vi "CAL-Interp (Fs, Npts).vi"(0 "Frequency (Hz)":dbl[](array[numeric]), 5 "Magnitude (dB)":dbl[](array[numeric]), 7 "Phase (degrees)":dbl[](array[numeric]), 9 "Fs (Hz)":dbl, 11 "Npts":i32) -> (4 "Interp Freq (Hz)":dbl[](array[numeric]), 6 "Interp Magnitude (dB)":dbl[](array[numeric]), 8 "Interp Phase (degrees)":dbl[](array[numeric]), 15 "Interp z":cdb[](array[numeric]))   [LabVIEW 2020]
uses:
  epl-vi-lib/Utility VIs/Math VIs/LinSpace (x0-dx-npts).vi
  918d1905-b6a0-4792-ae90-c7ddb557a04e.vi
  134e58aa-5bf1-43ce-a1c6-9a5bd50e3390.vi
  e1cc8427-bc3c-4687-9115-91c34d18d393.vi
  <vilib>/gmath/NI_Gmath.lvlib
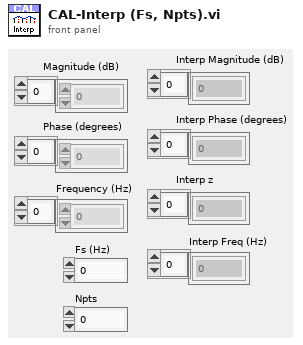
[diagram p1: front panel]
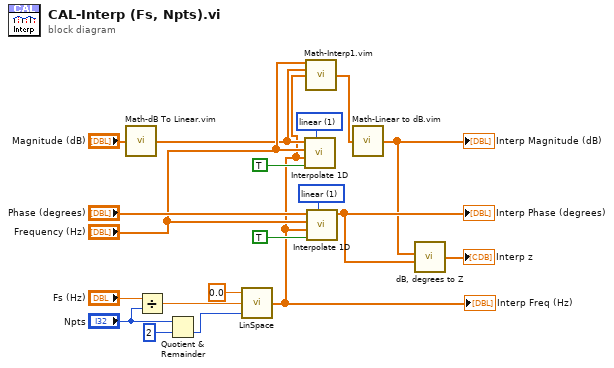
[diagram p0: block diagram]
diagram:
  w16 = 1 items=["nearest", "linear", "spline", "cubic Hermite", "Lagrange"] ("method")
  w19 = 1 items=["nearest", "linear", "spline", "cubic Hermite", "Lagrange"] ("method")
  n1 = call "Math-dB To Linear.vim"("dB"="Magnitude (dB)") -> ("linear"=w8:dbl[])
  n2 = Divide(x="Fs (Hz)", y="Npts") -> (x/y=w4:dbl)
  n3 = Quotient & Remainder(x="Npts", y=2) -> (floor(x/y)=w1:i32)  [unwired: 1 out]
  n4 = call-poly "LinSpace.vi"("npts"=w1, "dx"=w4, "x0"=0.0 ("Start")) -> ("Array"=w7:dbl[])  [unwired: 1 in, 1 out]
  "Interp Freq (Hz)" <- w7
  n5 = call <vilib>:"Interpolate 1D.vi"("method"=w19, "X is monotonic"=TRUE, "xi"=w7, "X"="Frequency (Hz)", "Y"=w8) -> ()  [unwired: 4 in, 3 out]
  n6 = call "Math-Interp1.vim"("X"="Frequency (Hz)", "Y"=w8, "U"=w7) -> ("V"=w6:dbl[])  [unwired: 12 in]
  n7 = call <vilib>:"Interpolate 1D.vi"("method"=w16, "X is monotonic"=TRUE, "xi"=w7, "X"="Frequency (Hz)", "Y"="Phase (degrees)") -> ("yi"=w13:dbl[])  [unwired: 4 in, 2 out]
  "Interp Phase (degrees)" <- w13
  n8 = call "Math-Linear to dB.vim"("linear"=w6) -> ("dB"=w11:dbl[])
  "Interp Magnitude (dB)" <- w11
  n9 = call "dB, degrees to Z.vi"("Magnitude (dB)"=w11, "Phase (degrees)"=w13) -> ("Z"=→"Interp z":cdb[])  [unwired: 5 in]
